vi "Update Post Test Actions.vi"(2 "Enable Slack Messaging?":bool=TRUE) -> ()   [LabVIEW 2013]
uses:
  <vilib>/Utility/config.llb/Write Key (Path).vi
  <vilib>/Utility/config.llb/Write Key (String).vi
  <vilib>/Utility/config.llb/Write Key (Boolean).vi
  <vilib>/Utility/config.llb/NI_LVConfig.lvlib
panel:
  out "Error Out":errorcluster
  in  "Cluster":T1={"Filename Keyword to Skip"="QuickView", "Destination Path Folder"=path "\\\\dfw0engfs02\\tld/DalCharData/Data/Incoming Data from Probers", "Test Station Folder"=path "C:/Users/cktesttx/Desktop/Test Data", "Text Message"="New data has been automatically posted to the \\\\\\\\dlfiles\\DalCharData\\Data\\Incoming Data from Probers\\ folder. Please copy data to your local machine to view", "Station Name"="Dinesh", "Channel"="dallas_lab", "Token Owner"="Eddie.Rickey", "Token"="xoxp-65464067636-73030412340-371308431078-00a7f651898a061f968f2e3bfb6c9d51"}
  in  "Error In":errorcluster
  # "SLACK Messaging"
  # "Station Information"
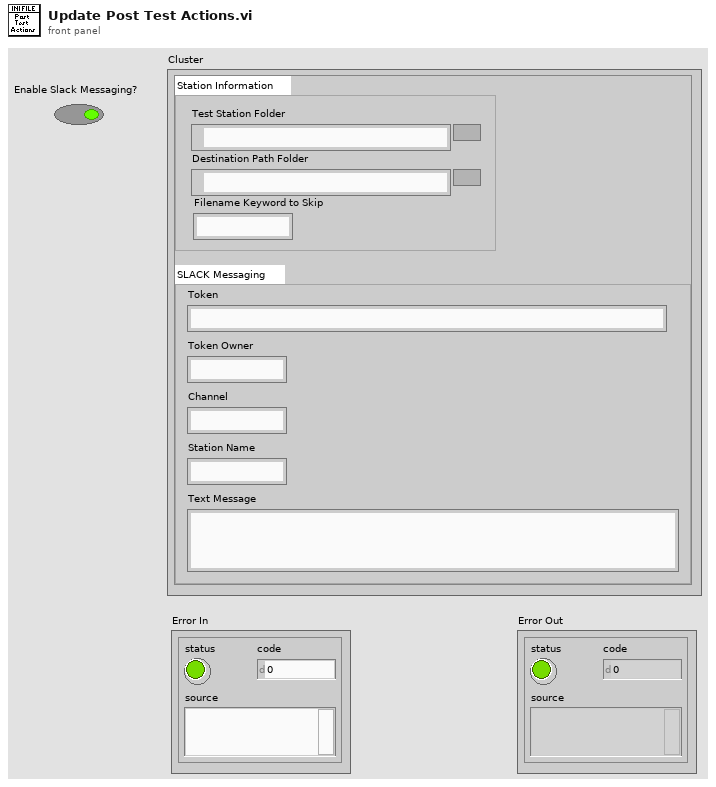
[diagram p1: front panel]
types:
  T1 = cluster{"Filename Keyword to Skip":string, "Destination Path Folder":path, "Test Station Folder":path, "Text Message":string, "Station Name":string, "Channel":string, "Token Owner":string, "Token":string}
  T2 = typedef "NI_LVConfig.lvlib/Config Data RefNum.ctl" = refnum<k1>
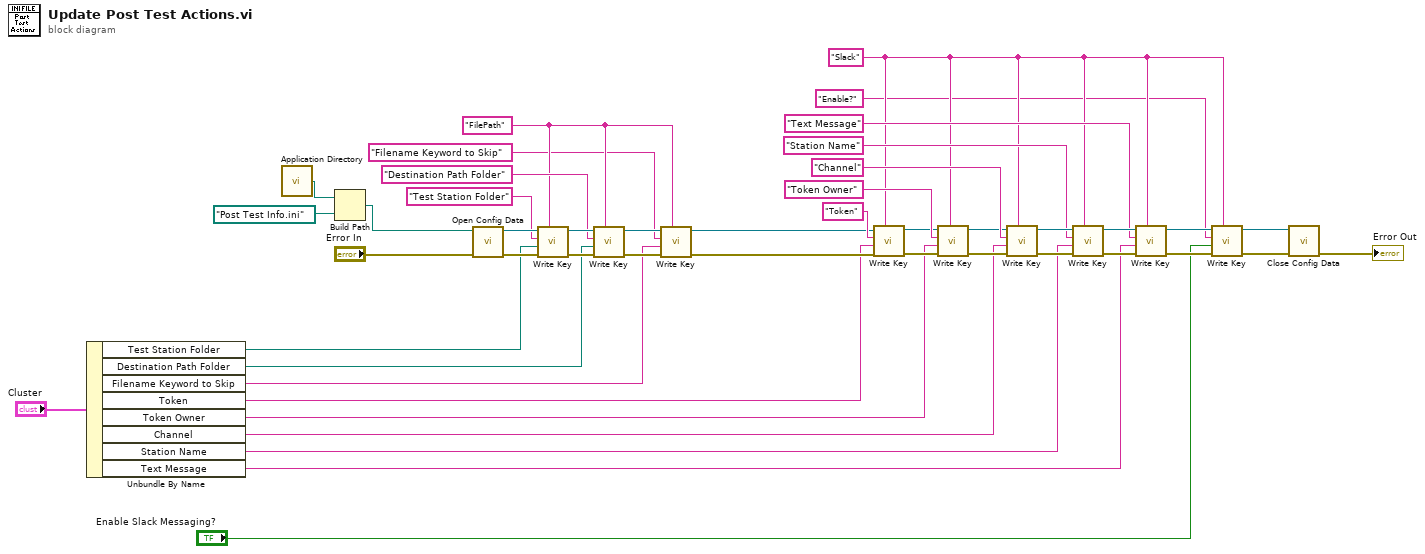
[diagram p0: block diagram]
diagram:
  w15 = "Slack" ("section")
  w34 = "FilePath" ("section")
  n1 = Unbundle By Name("Cluster") -> ("Test Station Folder"=w10:path, "Destination Path Folder"=w9:path, "Filename Keyword to Skip"=w8:string, "Token"=w7:string, "Token Owner"=w6:string, "Channel"=w5:string, "Station Name"=w4:string, "Text Message"=w3:string)
  n2 = call <vilib>:"Application Directory.vi"() -> ("Application Directory"=w45:path)
  n3 = Build Path(base path=w45, name or relative path=path "Post Test Info.ini" ("default name")) -> (appended path=w44:path)
  n4 = call <vilib>:"Open Config Data.vi"("error in (no error)"="Error In", "configuration file path"=w44) -> ("error out"=w41:errorcluster, "refnum"=w42:T2)  [unwired: 7 in, 1 out]
  n5 = call-poly <vilib>:"Write Key.vi"("section"=w34, "error in (no error)"=w41, "value"=w10, "key"="Test Station Folder", "refnum"=w42) -> ("error out"=w39:errorcluster, "refnum out"=w38:T2)  [unwired: 4 in, 1 out]
  n6 = call-poly <vilib>:"Write Key.vi"("section"=w34, "error in (no error)"=w39, "value"=w9, "key"="Destination Path Folder", "refnum"=w38) -> ("error out"=w36:errorcluster, "refnum out"=w35:T2)  [unwired: 4 in, 1 out]
  n7 = call-poly <vilib>:"Write Key.vi"("section"=w34, "error in (no error)"=w36, "value"=w8, "key"="Filename Keyword to Skip", "refnum"=w35) -> ("error out"=w28:errorcluster, "refnum out"=w24:T2)  [unwired: 4 in, 1 out]
  n8 = call-poly <vilib>:"Write Key.vi"("section"=w15, "error in (no error)"=w28, "value"=w7, "key"="Token", "refnum"=w24) -> ("error out"=w32:errorcluster, "refnum out"=w23:T2)  [unwired: 4 in, 1 out]
  n9 = call-poly <vilib>:"Write Key.vi"("section"=w15, "error in (no error)"=w32, "value"=w6, "key"="Token Owner", "refnum"=w23) -> ("error out"=w31:errorcluster, "refnum out"=w22:T2)  [unwired: 4 in, 1 out]
  n10 = call-poly <vilib>:"Write Key.vi"("section"=w15, "error in (no error)"=w31, "value"=w5, "key"="Channel", "refnum"=w22) -> ("error out"=w30:errorcluster, "refnum out"=w21:T2)  [unwired: 4 in, 1 out]
  n11 = call-poly <vilib>:"Write Key.vi"("section"=w15, "error in (no error)"=w30, "value"=w4, "key"="Station Name", "refnum"=w21) -> ("error out"=w29:errorcluster, "refnum out"=w20:T2)  [unwired: 4 in, 1 out]
  n12 = call-poly <vilib>:"Write Key.vi"("section"=w15, "error in (no error)"=w29, "value"=w3, "key"="Text Message", "refnum"=w20) -> ("error out"=w17:errorcluster, "refnum out"=w16:T2)  [unwired: 4 in, 1 out]
  n13 = call-poly <vilib>:"Write Key.vi"("section"=w15, "error in (no error)"=w17, "value"="Enable Slack Messaging?", "key"="Enable?", "refnum"=w16) -> ("error out"=w13:errorcluster, "refnum out"=w14:T2)  [unwired: 4 in, 1 out]
  n14 = call <vilib>:"Close Config Data.vi"("error in (no error)"=w13, "refnum"=w14) -> ("error out"=→"Error Out":errorcluster)  [unwired: 8 in, 1 out]
